vi "fgt read Ttl.vi"(8 "error in (no error)":errorcluster, 11 "TtlIndex":u32) -> (0 "error out":errorcluster, 3 "state out":bool)   [LabVIEW 2016, in "fgt_SDK.lvlib"]
doc: "Read TTL ports (BNC ports) if set as input."
uses:
  fgt_SDK.lvlib
  dlls/fgt_SDK_32.dll
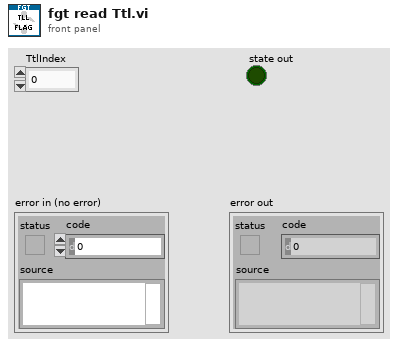
[diagram p1: front panel]
types:
  T1 = typedef "fgt_SDK.lvlib/fgt_STATUS_INFO.ctl" = cluster{"InstrType":T2, "instrSN":u16, "errorCode":u8, "infoCode":u8, "detail":string}
  T2 = typedef "fgt_SDK.lvlib/fgt_INSTRUMENT_TYPE.ctl" = enum32{"None", "MFCS", "MFCS_EZ", "FRP", "LineUP"}
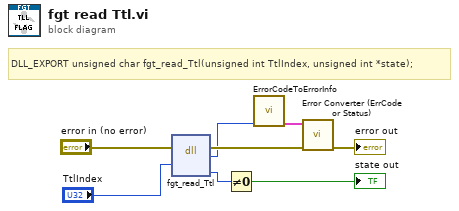
[diagram p0: block diagram]
diagram:
  # "DLL_EXPORT unsigned char fgt_read_Ttl(unsigned int TtlIndex, unsigned int *state);"
  n1 = dll-call lib="PTH2Zabs D\nMes DocumentsDéveloppementFluigentSDKsfgt-sdk-labviewdllsfgt_SDK_*.*" fn="fgt_read_Ttl"(error in="error in (no error)", "TtlIndex"="TtlIndex") -> (error out=w5:errorcluster, "return type"=w3:u8, "state"=w7:u32)  [unwired: 4 in, 1 out]
  n2 = Not Equal To 0?(x=w7) -> (x != 0?=→"state out":bool)
  n3 = call "ErrorCodeToErrorInfo.vi"("return type"=w3) -> ("StatusInfo"=w2:T1)  [unwired: 10 in]
  n4 = call "Error Converter (ErrCode or Status).vi"("error in (no error)"=w5, "StatusInfo"=w2) -> ("error out"=→"error out":errorcluster)  [unwired: 9 in]
